vi "Get Role.vi"(11 "User Data":refnum<class "User.lvclass">) -> (3 "Role":T1)   [LabVIEW 2026, in "User.lvclass"]
uses:
  User.lvclass
  User.lvclass/User.ctl
  Typedefs/enums/Role Enum.ctl
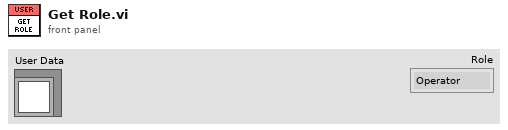
[diagram p1: front panel]
types:
  T1 = typedef "Role Enum.ctl" = enum16{"Operator", "Engineer", "Admin"}
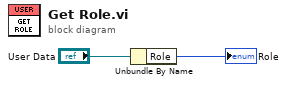
[diagram p0: block diagram]
diagram:
  n1 = Unbundle By Name("User Data") -> ("Role"=→"Role":T1)
